vi "CounterStuff2.vi"() -> ()   [LabVIEW 2012]
uses:
  <vilib>/DAQmx/write.llb/DAQmx Write (Analog 1D DBL 1Chan NSamp).vi
  <vilib>/DAQmx/create/channels.llb/DAQmx Create Channel (CO-Pulse Generation-Frequency).vi
  <vilib>/DAQmx/configure/timing.llb/DAQmx Timing (Implicit).vi
  <vilib>/DAQmx/create/channels.llb/DAQmx Create Channel (AO-Voltage-Basic).vi
  <vilib>/DAQmx/configure/timing.llb/DAQmx Timing (Sample Clock).vi
  <vilib>/DAQmx/miscellaneous.llb/DAQmx Fill In Error Info.vi
panel:
  in  "stop":bool
  in  "Pixels (Lines)":dbl=256.0
  in  "Pixeltime (ms)":dbl=1.0
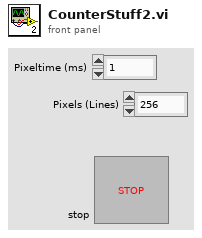
[diagram p1: front panel]
types:
  T1 = cluster{"task out":refnum<k21>, "task out":refnum<k21>, "task out":refnum<k21>, "task out":refnum<k21>, "task out":refnum<k21>}
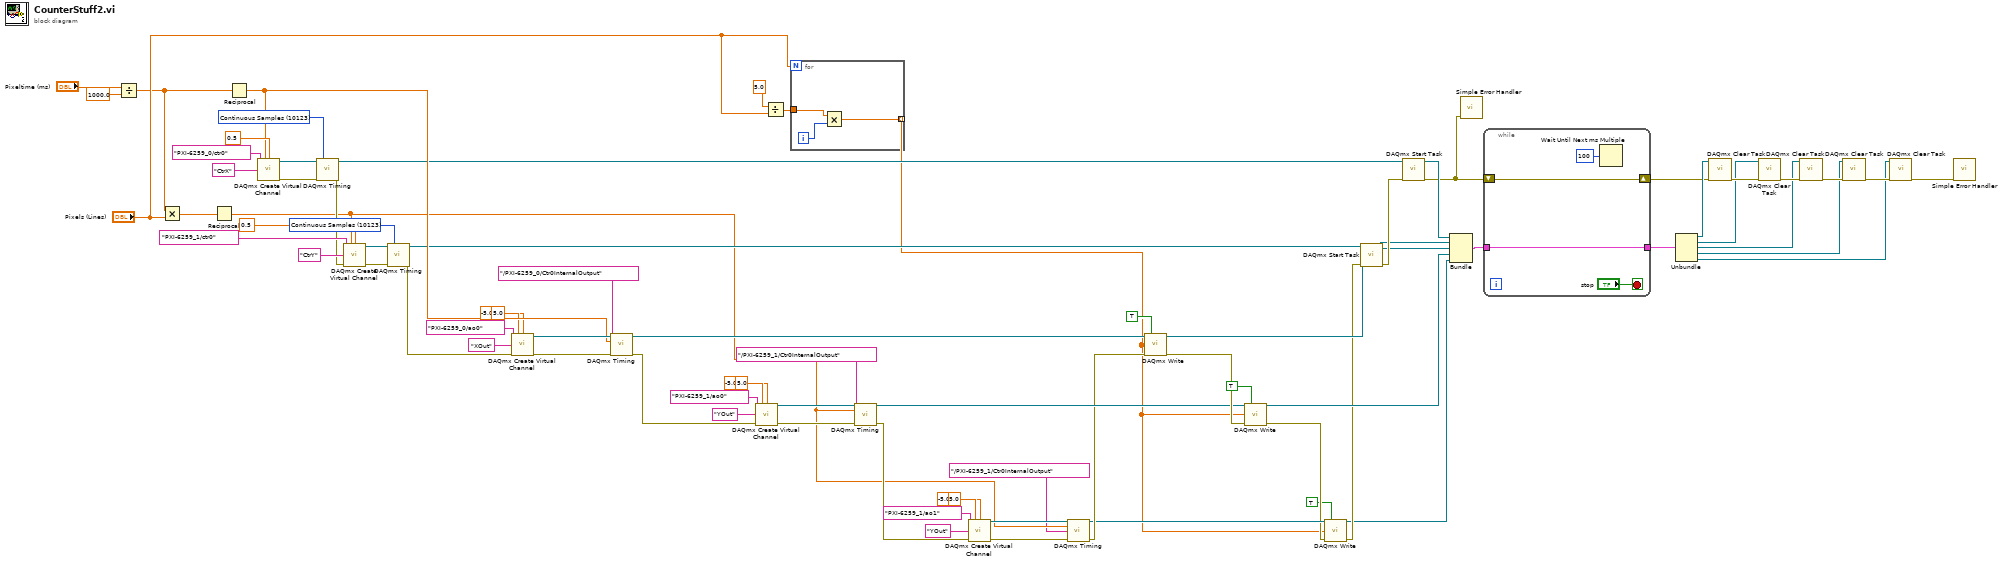
[diagram p0: block diagram]
diagram:
  w21 = 10123 items=["Finite Samples"=10178, "Continuous Samples"=10123, "Hardware Timed Single Point"=12522] ("sample mode")
  w25 = 10123 items=["Finite Samples"=10178, "Continuous Samples"=10123, "Hardware Timed Single Point"=12522] ("sample mode")
  n1 = Divide(x="Pixeltime (ms)", y=1000.0) -> (x/y=w38:dbl)
  n2 = Multiply(x=w38, y="Pixels (Lines)") -> (x*y=w76:dbl)
  n3 = Reciprocal(x=w76) -> (1/x=w11:dbl)
  n4 = Reciprocal(x=w38) -> (1/x=w71:dbl)
  n5 = call-poly <vilib>:"DAQmx Create Virtual Channel.vi"("frequency"=w71, "duty cycle"=0.5, "counter"=tag "PXI-6259_0/ctr0", "name to assign"="CtrX") -> ("task out"=w28:refnum<k21>, "error out"=w29:errorcluster)  [unwired: 10 in]
  n6 = call-poly <vilib>:"DAQmx Timing.vi"("task/channels in"=w28, "sample mode"=w25, "error in"=w29) -> ("task out"=w27:refnum<k21>, "error out"=w26:errorcluster)  [unwired: 11 in]
  n7 = call-poly <vilib>:"DAQmx Create Virtual Channel.vi"("frequency"=w11, "duty cycle"=0.5, "counter"=tag "PXI-6259_1/ctr0", "name to assign"="CtrY", "error in"=w26) -> ("task out"=w24:refnum<k21>, "error out"=w22:errorcluster)  [unwired: 9 in]
  n8 = call-poly <vilib>:"DAQmx Timing.vi"("task/channels in"=w24, "sample mode"=w21, "error in"=w22) -> ("task out"=w23:refnum<k21>, "error out"=w20:errorcluster)  [unwired: 11 in]
  n9 = call-poly <vilib>:"DAQmx Create Virtual Channel.vi"("maximum value"=5.0, "minimum value"=-5.0, "physical channels"=tag "PXI-6259_0/ao0", "name to assign"="XOut", "error in"=w20) -> ("task out"=w72:refnum<k21>, "error out"=w73:errorcluster)  [unwired: 9 in]
  n10 = call-poly <vilib>:"DAQmx Timing.vi"("task/channels in"=w72, "rate"=w71, "source"=tag "/PXI-6259_0/Ctr0InternalOutput", "error in"=w73) -> ("task out"=w66:refnum<k21>, "error out"=w69:errorcluster)  [unwired: 10 in]
  n11 = call-poly <vilib>:"DAQmx Create Virtual Channel.vi"("maximum value"=5.0, "minimum value"=-5.0, "physical channels"=tag "PXI-6259_1/ao0", "name to assign"="YOut", "error in"=w69) -> ("task out"=w67:refnum<k21>, "error out"=w70:errorcluster)  [unwired: 9 in]
  n12 = Divide(x=5.0, y="Pixels (Lines)") -> (x/y=w57:dbl)
  n13 = for {
    N: "Pixels (Lines)" -> [_]
    tunnel: w57 -> [w82]
    tunnel: [w80] -> w5 mode=indexing
    i -> [w81]
    n14 = Multiply(x=w82, y=w81) -> (x*y=w80:dbl)
  }
  n15 = call-poly <vilib>:"DAQmx Timing.vi"("task/channels in"=w67, "rate"=w11, "source"=tag "/PXI-6259_1/Ctr0InternalOutput", "error in"=w70) -> ("task out"=w64:refnum<k21>, "error out"=w13:errorcluster)  [unwired: 10 in]
  n16 = call-poly <vilib>:"DAQmx Create Virtual Channel.vi"("maximum value"=5.0, "minimum value"=-5.0, "physical channels"=tag "PXI-6259_1/ao1", "name to assign"="YOut", "error in"=w13) -> ("task out"=w17:refnum<k21>, "error out"=w19:errorcluster)  [unwired: 9 in]
  n17 = call-poly <vilib>:"DAQmx Timing.vi"("task/channels in"=w17, "rate"=w11, "source"=tag "/PXI-6259_1/Ctr0InternalOutput", "error in"=w19) -> ("task out"=w9:refnum<k21>, "error out"=w12:errorcluster)  [unwired: 10 in]
  n18 = call-poly <vilib>:"DAQmx Write.vi"("task/channels in"=w66, "auto start"=TRUE, "data"=w5, "error in"=w12) -> ("task out"=w51:refnum<k21>, "error out"=w65:errorcluster)  [unwired: 9 in, 1 out]
  n19 = call-poly <vilib>:"DAQmx Write.vi"("task/channels in"=w64, "auto start"=TRUE, "data"=w5, "error in"=w65) -> ("task out"=w50:refnum<k21>, "error out"=w8:errorcluster)  [unwired: 9 in, 1 out]
  n20 = call-poly <vilib>:"DAQmx Write.vi"("task/channels in"=w9, "auto start"=TRUE, "data"=w5, "error in"=w8) -> ("task out"=w4:refnum<k21>, "error out"=w7:errorcluster)  [unwired: 9 in, 1 out]
  n21 = call <vilib>:"DAQmx Start Task.vi"("task/channels in"=w23, "error in"=w7) -> ("task out"=w52:refnum<k21>, "error out"=w54:errorcluster)  [unwired: 12 in]
  n22 = call <vilib>:"DAQmx Start Task.vi"("task/channels in"=w27, "error in"=w54) -> ("task out"=w53:refnum<k21>, "error out"=w36:errorcluster)  [unwired: 12 in]
  n23 = Bundle("task out"=w53, "task out"=w52, "task out"=w51, "task out"=w50, "task out"=w4) -> (w49:T1)  [unwired: 1 in]
  n24 = call <vilib>:"Simple Error Handler.vi"("error in (no error)"=w36) -> ()  [unwired: 4 in, 5 out]
  n25 = while {
    tunnel: w49 -> [w84]
    shift-right: [w85] -> w40
    shift-left: w36 -> [w85]
    tunnel: [w84] -> w48
    stop <- "stop" stop-if-true
    n26 = Wait Until Next ms Multiple(millisecond multiple=u32 100) -> ()  [unwired: 1 out]
  }
  n27 = Unbundle(w48) -> ("task out"=w47:refnum<k21>, "task out"=w45:refnum<k21>, "task out"=w43:refnum<k21>, "task out"=w41:refnum<k21>, "task out"=w2:refnum<k21>)
  n28 = call <vilib>:"DAQmx Clear Task.vi"("task in"=w47, "error in"=w40) -> ("error out"=w46:errorcluster)  [unwired: 13 in]
  n29 = call <vilib>:"DAQmx Clear Task.vi"("task in"=w45, "error in"=w46) -> ("error out"=w44:errorcluster)  [unwired: 13 in]
  n30 = call <vilib>:"DAQmx Clear Task.vi"("task in"=w43, "error in"=w44) -> ("error out"=w42:errorcluster)  [unwired: 13 in]
  n31 = call <vilib>:"DAQmx Clear Task.vi"("task in"=w41, "error in"=w42) -> ("error out"=w3:errorcluster)  [unwired: 13 in]
  n32 = call <vilib>:"DAQmx Clear Task.vi"("task in"=w2, "error in"=w3) -> ("error out"=w1:errorcluster)  [unwired: 13 in]
  n33 = call <vilib>:"Simple Error Handler.vi"("error in (no error)"=w1) -> ()  [unwired: 4 in, 5 out]
